vi "calculate_average.vi"(4 "error in":errorcluster={"status"=FALSE, "code"=0, "source"="Event Code: 0\r\ncomplete\r\n-----------------------------------\nEvent Code: 0\r\ncomplete\r\n-----------------------------------\nEvent Code: 0\r\nweather configured to \"Default\"\r\n-----------------------------------\nEvent Code: 0\r\ncomplete\r\n-----------------------------------\nEvent Code: 0\r\nsimulator configuration mode = 1\r\n-----------------------------------\nEvent Code: 0\r\nsimulator_version: 1.10.0, api_version: 3.0\r\n-----------------------------------\nEvent Code: 0\r\n\r\n-----------------------------------\n"}, 7 "Values to average":sgl[](array[numeric])) -> (0 "error out":errorcluster={"status"=FALSE, "code"=0, "source"="Event Code: 0\r\ncomplete\r\n-----------------------------------\nEvent Code: 0\r\ncomplete\r\n-----------------------------------\nEvent Code: 0\r\nweather configured to \"Default\"\r\n-----------------------------------\nEvent Code: 0\r\ncomplete\r\n-----------------------------------\nEvent Code: 0\r\nsimulator configuration mode = 1\r\n-----------------------------------\nEvent Code: 0\r\nsimulator_version: 1.10.0, api_version: 3.0\r\n-----------------------------------\nEvent Code: 0\r\n\r\n-----------------------------------\n"}, 3 "Average":sgl)   [LabVIEW 2019]
doc: "Calculate the average for the given input array of values"
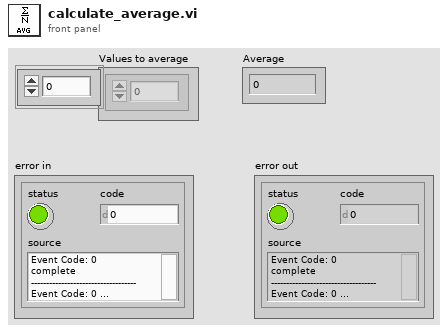
[diagram p1: front panel]
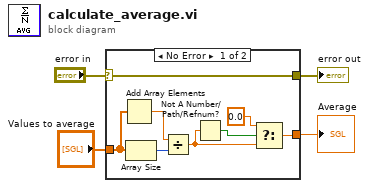
[diagram p0: block diagram]
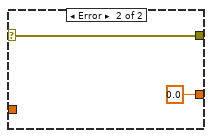
[diagram p2: hidden frame]
diagram:
  n1 = case shown="No Error" "error in" {
    selector: "error in" -> [w5 w13]
    tunnel: [w12 0.0 ("t")] -> w4
    tunnel: "Values to average" -> [w11 _]
    tunnel: [w5 w13] -> w1
    frame No Error {
      n2 = Add Array Elements(numeric array=w11) -> (sum=w8:sgl)
      n3 = Array Size(array=w11) -> (size(s)=w9:i32)
      n4 = Divide(x=w8, y=w9) -> (x/y=w6:sgl)
      n5 = Not A Number/Path/Refnum?(number/path/refnum=w6) -> (NaN/Path/Refnum?=w7:bool)
      n6 = Select(t=0.0, s=w7, f=w6) -> (s? t:f=w12:dbl)
    }
    frame Error {
    }
  }
  "Average" <- w4
  "error out" <- w1
